vi "populate.vi"() -> ()   [LabVIEW 2021]
uses:
  build/test/libtest.so
panel:
  out "error out":errorcluster
  in  "array":i32[](array[numeric])=[1, 2, 3]
  out "Resized Array":i32[](array[numeric])=[2, 4, 6, 8]
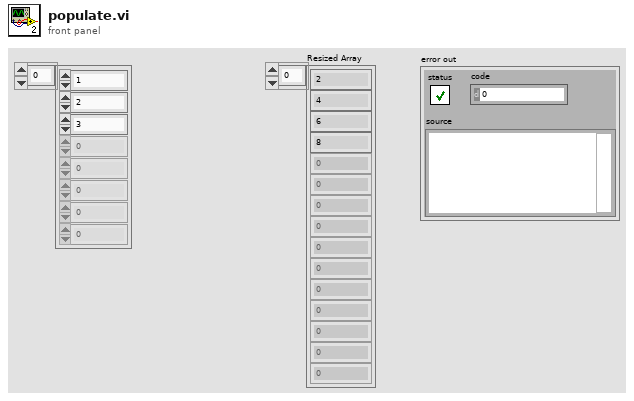
[diagram p1: front panel]
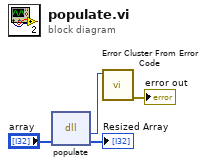
[diagram p0: block diagram]
diagram:
  n1 = dll-call lib="home/saman/src/lvcc/build/test/libtest.so" fn="populate"("arr"="array") -> ("return type"=w2:i32, "arr"=→"Resized Array":i32[])  [unwired: 3 in, 2 out]
  n2 = call <vilib>:"Error Cluster From Error Code.vi"("error code (0)"=w2) -> ("error out"=→"error out":errorcluster)  [unwired: 8 in]
